vi "Initialize.vi"(8 "error in (no error)":errorcluster, 11 "Test Configs In":T1) -> (0 "error out":errorcluster, 3 "Test Configs Out":T1)   [LabVIEW 2015]
doc: "Load the sequence parameters array with a single default element."
uses:
  Type Defs/Sequence Parameters Ref.ctl
  Type Defs/Sequence Parameters.ctl
  Type Defs/Target Type.ctl
  Type Defs/Variable Data Type.ctl
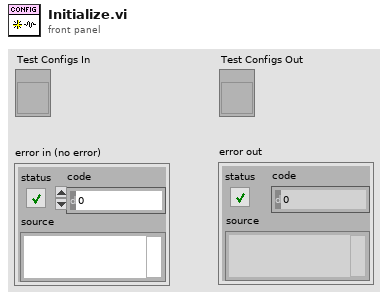
[diagram p1: front panel]
types:
  T1 = typedef "Sequence Parameters Ref.ctl" = refnum<vi>
  T2 = typedef "Sequence Parameters.ctl" = cluster{"Test Name":string, "Target":T3, "Host IP Address":string, "Target IP Address":string, "Shared Variable Host":enum16{"Target", "Host"}, "Shared Variable Writer":enum16{"Target", "Host"}, "Variable Data Type":T4, "# of Variables per Library":u16, "Update Rate (Hz)":dbl, "Read Rate (Hz)":dbl, "Floor":u32, "Ceiling":u32, "Delta":u32}
  T3 = typedef "Target Type.ctl" = enum16{"cRIO-9012", "cRIO-9014", "cRIO-9022", "cRIO-9023", "cRIO-9024", "cRIO-9025", "cRIO-9068", "cRIO-9073", "cRIO-9074", "cRIO-9075", "cRIO-9076", "cRIO-9081", "cRIO-9082", "myRIO-1900", "myRIO-1950", "PXI-8101", "PXI-8115", "PXI-8119", "PXI-8820", "PXIe-8100", "PXIe-8101", "PXIe-8133", "PXIe-8135", "PXIe-8820", "sbRIO-9605", "sbRIO-9606", "sbRIO-9623", "sbRIO-9626", "sbRIO-9633", "sbRIO-9636", "Unlisted (Linux-RT)", "Unlisted (PharLap)", "Unlisted (VxWorks)", "Windows Target"}
  T4 = typedef "Variable Data Type.ctl" = enum16{"U8", "U16", "U32", "U64", "I8", "I16", "I32", "I64", "Single", "Double", "Boolean", "String"}
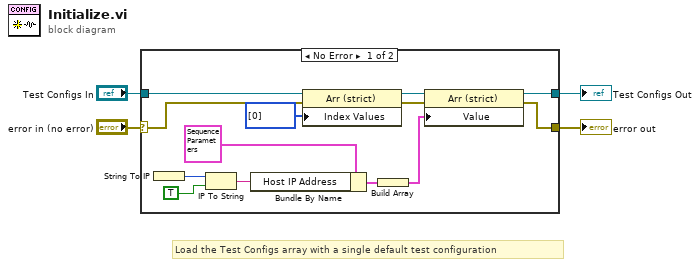
[diagram p0: block diagram]
diagram:
  # "Load the Test Configs array with a single default test configuration"
  n1 = case shown="No Error" "error in (no error)" {
    selector: "error in (no error)" -> [w6 w18]
    tunnel: "Test Configs In" -> [w9 w19]
    tunnel: [w17 w19] -> w1
    tunnel: [w16 w18] -> w3
    frame No Error {
      n2 = String To IP() -> (0:w13:u32)  [unwired: 1 in]
      n3 = IP To String(1:TRUE ("dot notation? (F)"), 2:w13) -> (0:w12:string)
      n4 = Bundle By Name(cluster=T2 {"Test Name"="Unique Test Name", "Target"=enum."cRIO-9012", "Host IP Address"="0.0.0.0", "Target IP Address"="0.0.0.0", "Shared Variable Host"=enum."Target", "Shared Variable Writer"=enum."Target", "Variable Data Type"=enum."Double", "# of Variables per Library"=500, "Update Rate (Hz)"=1.0, "Read Rate (Hz)"=1.0, "Floor"=500, "Ceiling"=5000, "Delta"=500} ("Test Parameters"), "Host IP Address"=w12) -> (w11:T2)
      n5 = property class="Arr (strict)"(reference=w9, error in=w6, "Index Values"=u32[] [0]) -> (reference out=w8:T1, error out=w7:errorcluster)
      n6 = Build Array(w11) -> (w10:T2[])
      n7 = property class="Arr (strict)"(reference=w8, error in=w7, "Value"=w10) -> (reference out=w17:T1, error out=w16:errorcluster)
    }
    frame Error {
    }
  }
  "error out" <- w3
  "Test Configs Out" <- w1
